vi "Add Prefix to Label.vi"(8 "error in (no error)":errorcluster, 10 "Prefix to add":string, 11 "Message":refnum<class "MSG.lvclass">) -> (0 "error out":errorcluster, 3 "Message":refnum<class "MSG.lvclass">)   [LabVIEW 2011, in "Messenging.lvlib" / "MSG.lvclass"]
uses:
  MSG.lvclass
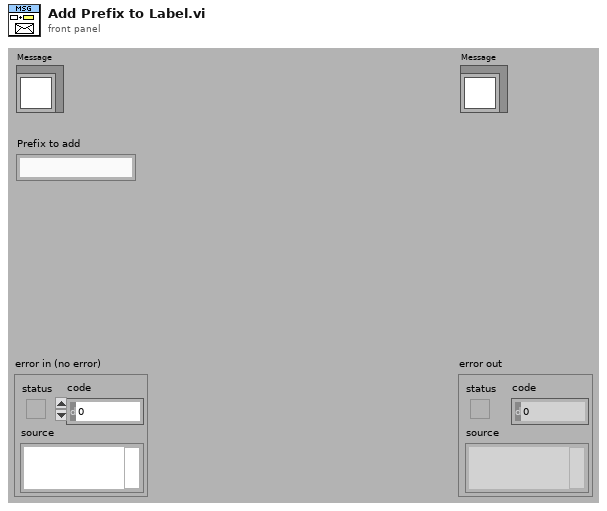
[diagram p1: front panel]
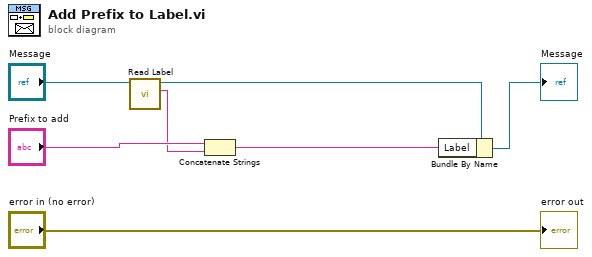
[diagram p0: block diagram]
diagram:
  n1 = call-dynamic "Read Label.vi"("Message"="Message") -> ("Label"=w1:string, "Message"=w3:refnum<class "MSG.lvclass">)  [unwired: 1 in, 8 out]
  n2 = Concatenate Strings("Prefix to add", w1) -> (w2:string)
  n3 = Bundle By Name(cluster=w3, "Label"=w2) -> (→"Message":refnum<class "MSG.lvclass">)
  "error out" <- "error in (no error)"
